vi "Ex9 Forward Fourier Transform.vi"() -> ()   [LabVIEW 2024]
uses:
  <vilib>/vision/Management.llb/Cast Image 2 Method.ctl
  <vilib>/vision/NI_Vision_Development_Module.lvlib
panel:
  in  "Color Plane":i32(ring)=1 items=["Red", "Green", "Blue", "Hue", "Saturation", "Luminance", "Value", "Intensity"]
  out "error out":errorcluster
  out "Color Channel":T1(plugin-control)
  out "Image":T1(plugin-control)
  in  "File Path":path
  # "EX.9 FORWARD FOURIER TRANSFORM"
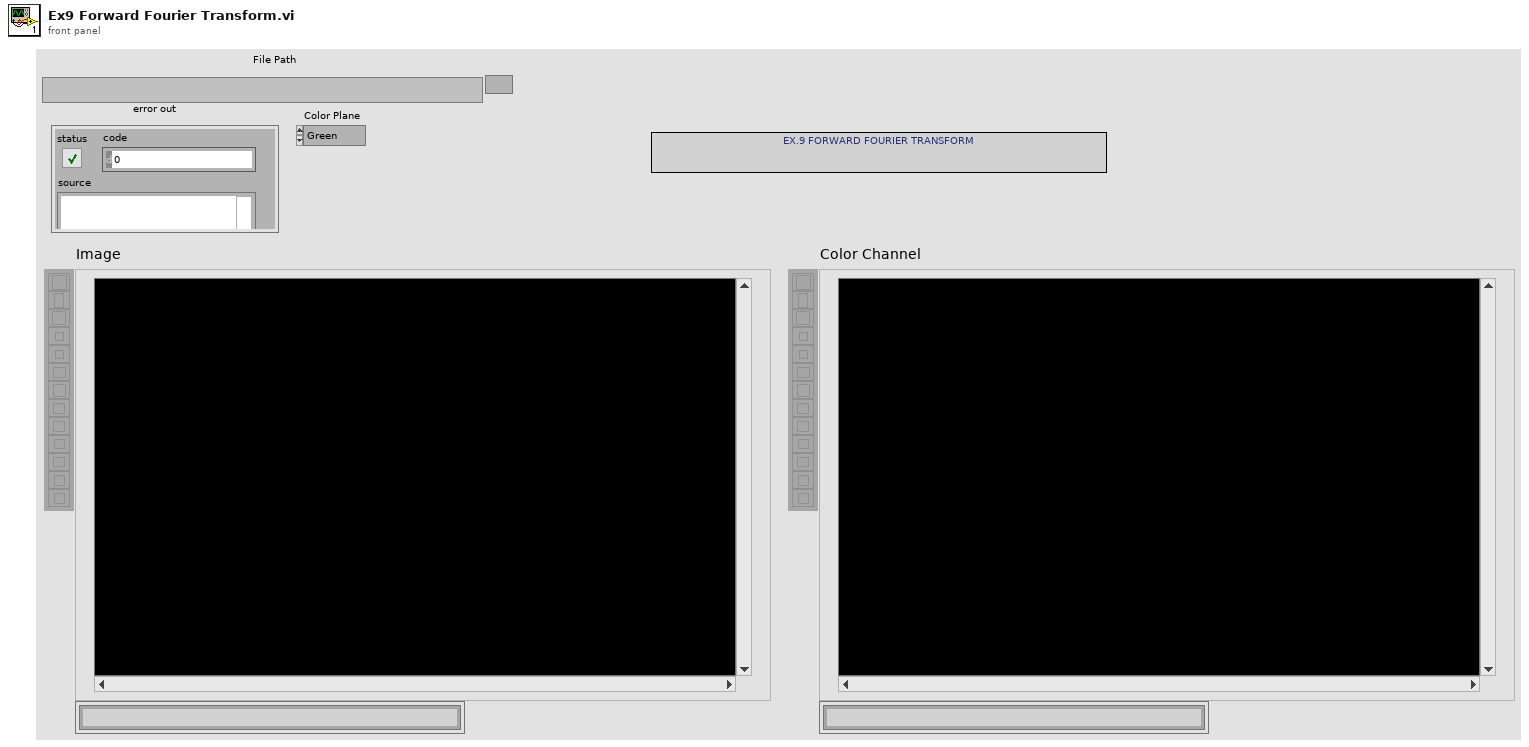
[diagram p1: front panel]
types:
  T1 = typedef "IMAQ Image.ctl" = refnum<image>
  T2 = typedef "Image Type" = u32
  T3 = typedef "Cast Image 2 Method.ctl" = u32
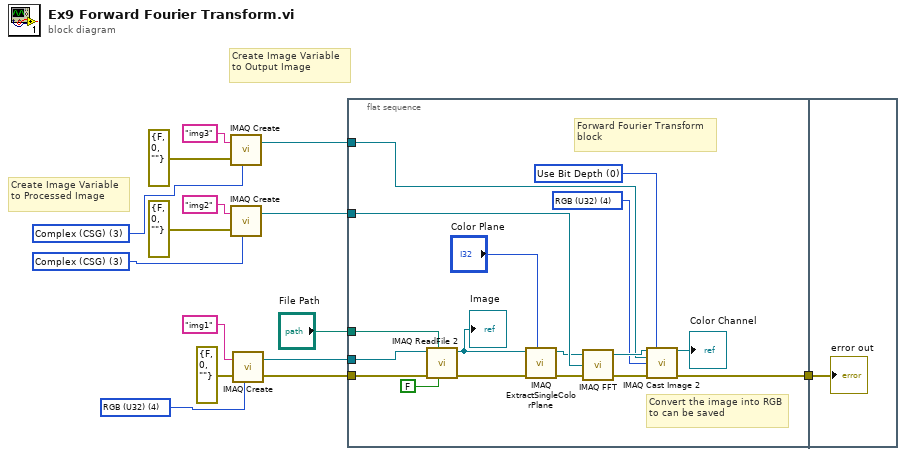
[diagram p0: block diagram]
diagram:
  w2 = T2 3 items=["Grayscale (U8)", "Grayscale (I16)", "Grayscale (SGL)", "Complex (CSG)", "RGB (U32)", "HSL (U32)", "RGB (U64)", "Grayscale (U16)"] ("Image Type")
  w5 = T2 4 items=["Grayscale (U8)", "Grayscale (I16)", "Grayscale (SGL)", "Complex (CSG)", "RGB (U32)", "HSL (U32)", "RGB (U64)", "Grayscale (U16)"] ("Image Type")
  w6 = T2 3 items=["Grayscale (U8)", "Grayscale (I16)", "Grayscale (SGL)", "Complex (CSG)", "RGB (U32)", "HSL (U32)", "RGB (U64)", "Grayscale (U16)"] ("Image Type")
  # "Create Image Variable to Processed Image"
  # "Create Image Variable to Output Image"
  n1 = call "IMAQ Create"("Image Name"="img3", "Image Type"=w2, "error in (no error)"=errorcluster {"status"=FALSE, "code"=0, "source"=""}) -> ("New Image"=w1:T1)  [unwired: 2 in, 1 out]
  n2 = call "IMAQ Create"("Image Name"="img2", "Image Type"=w6, "error in (no error)"=errorcluster {"status"=FALSE, "code"=0, "source"=""}) -> ("New Image"=w7:T1)  [unwired: 2 in, 1 out]
  n3 = call "IMAQ Create"("Image Name"="img1", "Image Type"=w5, "error in (no error)"=errorcluster {"status"=FALSE, "code"=0, "source"=""}) -> ("New Image"=w8:T1, "error out"=w9:errorcluster)  [unwired: 2 in]
  n4 = flat-sequence {
    tunnel: "File Path" -> [w31]
    tunnel: w9 -> [w30]
    tunnel: w8 -> [w29]
    tunnel: w7 -> [w28]
    tunnel: [w19] -> w15
    tunnel: w1 -> [w17]
    tunnel: w15 -> [w33]
    frame #0 {
      w16 = T2 4 items=["Grayscale (U8)", "Grayscale (I16)", "Grayscale (SGL)", "Complex (CSG)", "RGB (U32)", "HSL (U32)", "RGB (U64)", "Grayscale (U16)"] ("Image Type")
      w21 = T3 0 items=["Use Bit Depth", "Shift", "Use Lookup Table"] ("Method")
      # "Convert the image into RGB to can be saved"
      # "Forward Fourier Transform block"
      n5 = call "IMAQ ReadFile 2"("Use File Path Image Type"=FALSE, "File Path"=w31, "error in (no error)"=w30, "Image"=w29) -> ("error out"=w26:errorcluster, "Image Out"=w27:T1)  [unwired: 3 in, 3 out]
      "Image" <- w27
      n6 = call "IMAQ ExtractSingleColorPlane"("Color Plane"="Color Plane", "error in (no error)"=w26, "Image Src"=w27) -> ("error out"=w23:errorcluster, "Image Dst Out"=w24:T1)  [unwired: 7 in]
      n7 = call "IMAQ FFT"("error in (no error)"=w23, "Image Dst"=w28, "Image Src"=w24) -> ("error out"=w22:errorcluster, "Image Dst Out"=w18:T1)  [unwired: 1 in]
      n8 = call "IMAQ Cast Image 2"("Image Src"=w18, "Method"=w21, "Image Dst"=w17, "Image Type"=w16, "error in (no error)"=w22) -> ("Image Dst Out"=→"Color Channel":T1, "error out"=w19:errorcluster)  [unwired: 9 in]
    }
    frame #1 {
      "error out" <- w33
    }
  }
